vi "Close Remote Panel Connections.vi"() -> ()   [LabVIEW 2009]
panel:
  in  "vi path":path
  out "Remote Panel Connections":T1(array[cluster])
  # "Run this VI embedded on a desktop PC \nor on a Real-Time target. This VI dissconnects \nall the remote front panels that are connected \nto the specified VI."
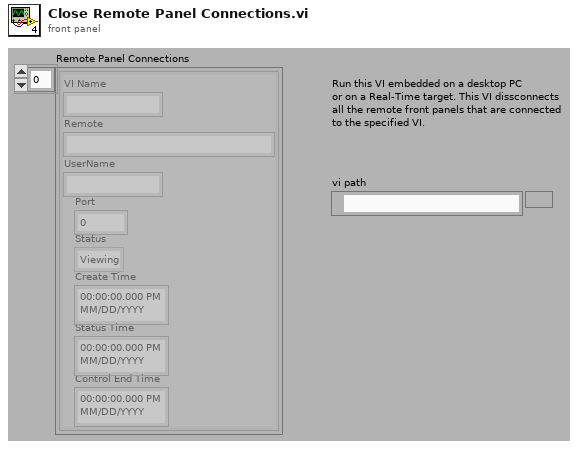
[diagram p1: front panel]
types:
  T1 = cluster{"VI Name":string, "Remote":string, "UserName":string, "Port":i32, "Status":enum32{"Viewing", "Waiting For Control", "Controlling"}, "Create Time":timestamp, "Status Time":timestamp, "Control End Time":timestamp}[]
  T2 = typedef "LVRemotePanelConnectionsTypeDef.ctl" = cluster{"VI Name":string, "Remote":string, "UserName":string, "Port":i32, "Status":enum32{"Viewing", "Waiting For Control", "Controlling"}, "Create Time":timestamp, "Status Time":timestamp, "Control End Time":timestamp}[]
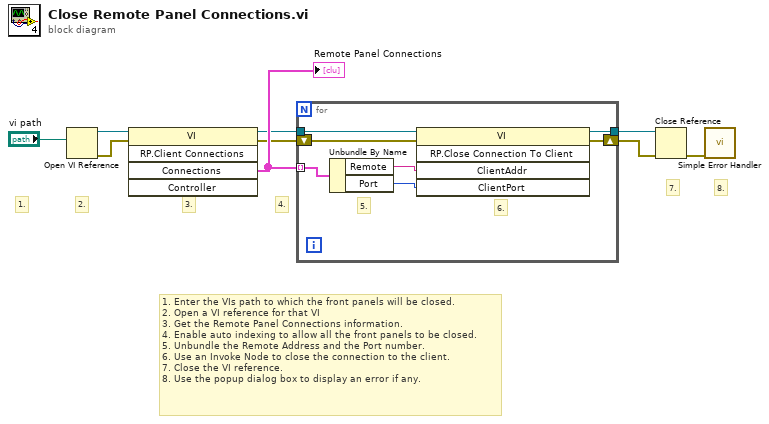
[diagram p0: block diagram]
diagram:
  # "8."
  # "7."
  # "4."
  # "3."
  # "2."
  # "1. Enter the VIs path to which the front panels will be closed.\n2. Open a VI reference for that VI\n3. Get the Remote Panel Connections information.\n4. Enable auto indexing to allow all the front panels to be closed.\n5. Unbundle the Remote Address and the Port number.\n6. Use an Invoke Node to close the connection to the client.\n7. Close the VI reference.\n8. Use the popup dialog box to display an error if any."
  # "1."
  n1 = Open VI Reference(vi path="vi path") -> (vi reference=w3:refnum<vi>, error out=w2:errorcluster)  [unwired: 5 in]
  n2 = invoke class="VI" method="RP.Client Connections"(reference=w3, error in=w2) -> (reference out=w8:refnum<vi>, error out=w7:errorcluster, "Connections"=w9:T2)  [unwired: 3 in, 2 out]
  "Remote Panel Connections" <- w9
  n3 = for {
    tunnel: w9 -> [w16] mode=indexing
    shift-right: [w12] -> w5
    shift-left: w7 -> [w14]
    tunnel: w8 -> [w15]
    tunnel: [w13] -> w6
    # "6."
    # "5."
    n4 = Unbundle By Name(w16) -> ("Remote"=w10:string, "Port"=w11:i32)
    n5 = invoke class="VI" method="RP.Close Connection To Client"(reference=w15, error in=w14, "ClientAddr"=w10, "ClientPort"=w11) -> (reference out=w13:refnum<vi>, error out=w12:errorcluster)  [unwired: 1 in, 3 out]
  }
  n6 = Close Reference(reference=w6, error in (no error)=w5) -> (error out=w4:errorcluster)
  n7 = call <vilib>:"Simple Error Handler.vi"("error in (no error)"=w4) -> ()  [unwired: 4 in, 5 out]
